vi "Global_ACT_Data Out.vi"() -> ()   [LabVIEW 2020, in "Cone_Stabber_ACT.lvlib"]
uses:
  ConeStabber/Cone_Stabber_ACT.lvlib
panel:
  out "ACT_Stabber_Level":bool
  out "ACT_Stabber_At Target":bool
  in  "ACT_Stabber_CycleTime(S)":dbl
  # "The Names of the Data items in the Global Variable MUST describe who the Single Writer is\nFor Actuator Globals the the naming convention is\n   \nACT_Lib Name_Data Name\n\nExamples:\nACT_Drive_X axis\nACT_Hopper_AgitatorSpeed"
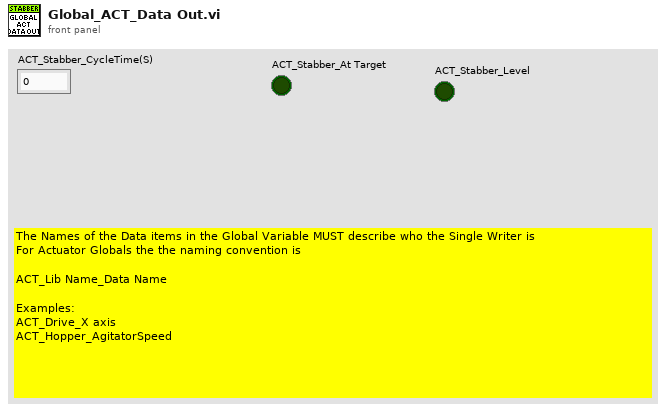
[diagram p1: front panel]
diagram:
